vi "I2C Lidar Present.vi"(8 "error in (no error)":errorcluster, 11 "I2CDevRef":T1 {"Device Address" format="%.0x"}) -> (3 "Sensor Present":bool)   [LabVIEW 2015]
uses:
  <vilib>/Rock Robotics/WPI/I2C/WPI_I2CDevRef.ctl
  <vilib>/Rock Robotics/SystemInterfaces/i2clib/i2c_bus.ctl
panel:
  out "Data Out":u8[](array[numeric])
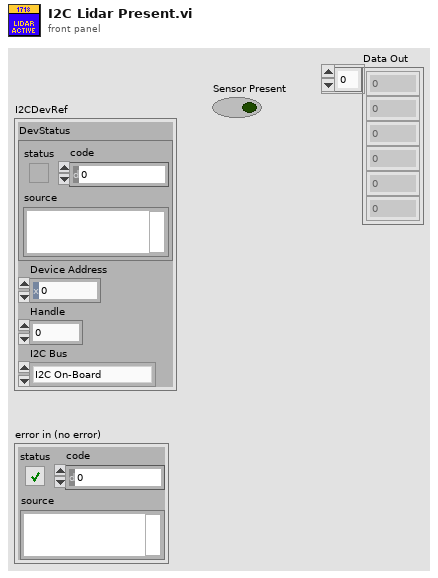
[diagram p1: front panel]
types:
  T1 = typedef "WPI_I2CDevRef.ctl" = cluster{"DevStatus":errorcluster, "Device Address":u8, "Handle":i32, "I2C Bus":T2}
  T2 = typedef "i2c_bus.ctl" = enum16{"I2C On-Board", "I2C MXP", "Invalid"}
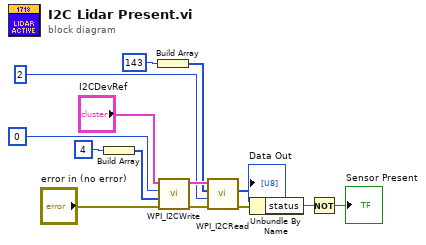
[diagram p0: block diagram]
diagram:
  n1 = Build Array(u8 4 ("Data To Send")) -> (w8:u8[])
  n2 = Build Array(u8 143 ("I2CRegister")) -> (w6:u8[])
  n3 = call <vilib>:"WPI_I2CWrite.vi"("error in (no error)"="error in (no error)", "I2CDataToSend"=w8, "I2CRegister"=u8 0 ("Data To Send"), "I2CDevRef"="I2CDevRef") -> ("error out"=w13:errorcluster, "I2CDevRef"=w7:T1)  [unwired: 6 out]
  n4 = call <vilib>:"WPI_I2CRead.vi"("error in (no error)"=w13, "I2CBytesToRead"=u8 2, "I2CRegister"=w6, "I2CDevRef"=w7) -> ("error out"=w14:errorcluster, "Data Out"=→"Data Out":u8[])  [unwired: 5 in, 1 out]
  n5 = Unbundle By Name(w14) -> ("status"=w3:bool)
  n6 = Not(x=w3) -> (.not. x?=→"Sensor Present":bool)
